vi "DCTOpticalSwitch.vi"() -> ()   [LabVIEW 2011]
uses:
  Dependencies/DCS/flex05-4chPascal.dll
  Dependencies/DCS/flex05oem8chautoPASCAL.dll
  Dependencies/Zaber/Zaber A Series.lvlib
panel:
  in  "Start Program":bool
  in  "DAQ Port":tag
  in  "Raster X Reverse":bool=TRUE
  in  "Max speed (mm/s)":dbl=35.0
  in  "Microstep resolution":dbl=0.124023437
  in  "Close":bool
  in  "Optical Output":T1
  in  "Optical Input":T2
  out "Detector Indicator":T3 {"Det 8" format="%.3f"; "Det 7" format="%.3f"; "Det 6" format="%.3f"; "Det 5" format="%.3f"; "Det 4" format="%.3f"; "Det 3" format="%.3f"; "Det 2 2" format="%.3f"; "Det 1" format="%.3f"}
  in  "Detector\n Buttons":T4
  out "Y-axis Device":string
  out "X-axis Device":string
  out "Y Index":i32
  out "X Index":i32
  in  "Update Time (ms):":u32=44
  out "Computer time":string
  out "Time Left (ms)":sgl format="%.3f"
  in  "Duration Time (ms):":sgl=2000.0
  out "Y Position [mm]":dbl
  out "X Position [mm]":dbl
  in  "Stage Controls Tabs":enum32{"Raster Scan", "Manual"}(tab) caption="Stage Controls"
  out "Raster Scanning":bool
  in  "X Steps":i32
  in  "Y Steps":i32
  in  "Y Increment [mm]":dbl
  in  "X Increment [mm]":dbl
  out "Y Total Distance [mm]":dbl
  out "X Total Distance [mm]":dbl
  in  "Raster Scan":bool
  out "Scanning":bool
  in  "Move X":bool
  in  "Move Y":bool
  in  "Home":bool
  in  "Scan":bool
  in  "Number of Scans":i32=1 min=1
  in  "X distance [mm]":dbl
  in  "Y distance  [mm]":dbl
  in  "File Name:":string="AAA"
  in  "File Path:":path=path "C:/Users/aproctor1/Desktop/Our Attempts/DCS practice data"
  in  "Clear Plots":bool
  out "g2":cluster{"Delay Time":sgl[], sgl[]}[](graph) caption="Normalized Correlation Function"
  out "Tau":T5(graph)={"[0]"=0.0, "[1]"=1.0, "[2]"=2.0, "[3]"=3.0, "[4]"=4.0, "[5]"=5.0, "[6]"=6.0, "[7]"=7.0, "[8]"=8.0} caption="Relative changes of flow"
  in  "Detectors Select":enum32{"4 Detectors", "8 Detectors"}(radio)
  in  "Stage Port":refnum<visa-resource-name>="COM8"
  # "DCS Control Panel"
  # "Optical Switch"
  # "Stage Control"
  # "Probe Location"
  # "Instructions: \n1. Initialize the following settings first: (these will be locked later)\n      - Detectors Select\n      - DAQ Port (port 0 for NI USB 6001)\n      - Optical Switch Inputs and Outputs\n      - Stage Port (for Zaber)\n2. Click on \"Start Program\" which will lock the above settings and enable stage controls\n3. When settings from step 1 are locked, input options for raster scanning or manual scanning\n4. Free to do whatever \n5. Close the program by clicking the close button"
  # "Max Distance: 203.2 mm"
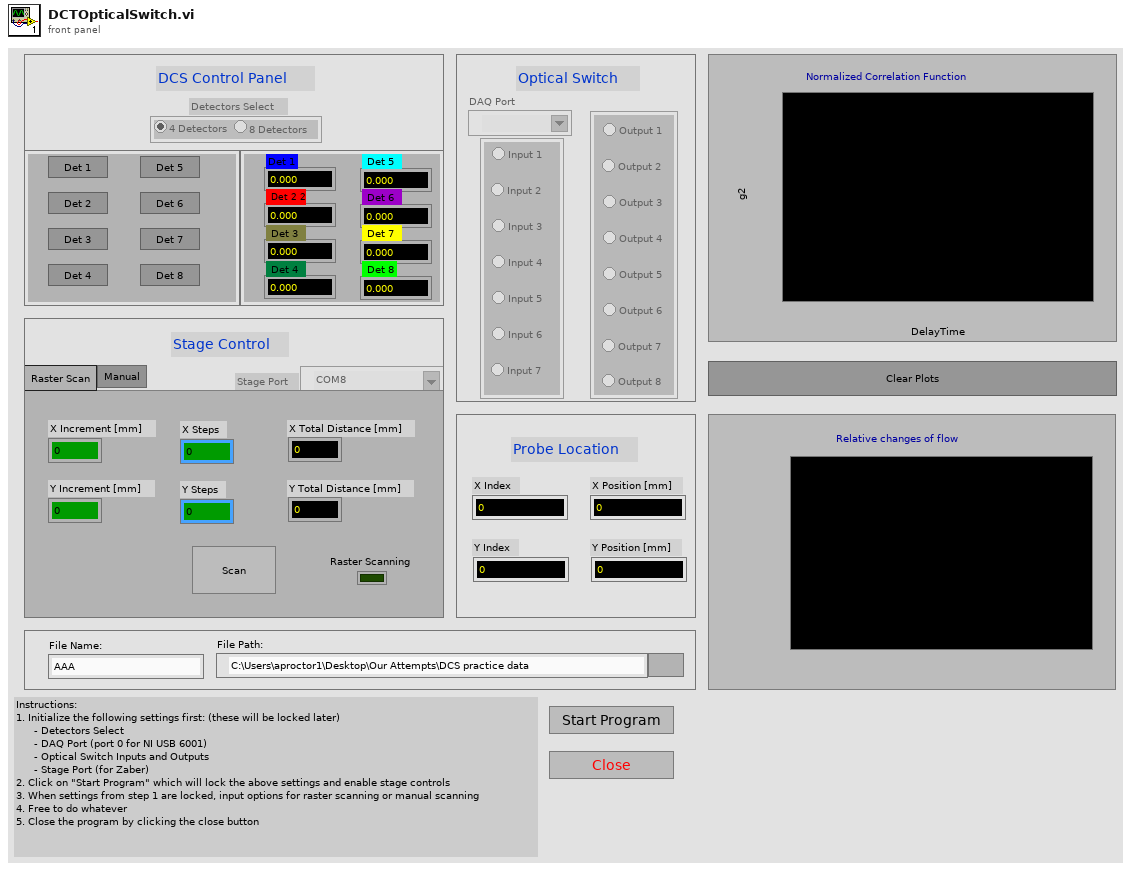
[diagram p1: front panel]
types:
  T1 = cluster{"Output 1":bool, "Output 2":bool, "Output 3":bool, "Output 4":bool, "Output 5":bool, "Output 6":bool, "Output 7":bool, "Output 8":bool}
  T2 = cluster{"Input 1":bool, "Input 2":bool, "Input 3":bool, "Input 4":bool, "Input 5":bool, "Input 6":bool, "Input 7":bool}
  T3 = cluster{"Det 1":sgl, " Det 2 2":sgl, " Det 3":sgl, " Det 4":sgl, " Det 5":sgl, " Det 6":sgl, " Det 7":sgl, " Det 8":sgl}
  T4 = cluster{"btnDet 1":bool, "btnDet 2":bool, "btnDet 3":bool, "btnDet 4":bool, "btnDet 5":bool, "btnDet 6":bool, "btnDet 7":bool, "btnDet 8":bool}
  T5 = cluster{"[0]":dbl, "[1]":dbl, "[2]":dbl, "[3]":dbl, "[4]":dbl, "[5]":dbl, "[6]":dbl, "[7]":dbl, "[8]":dbl}
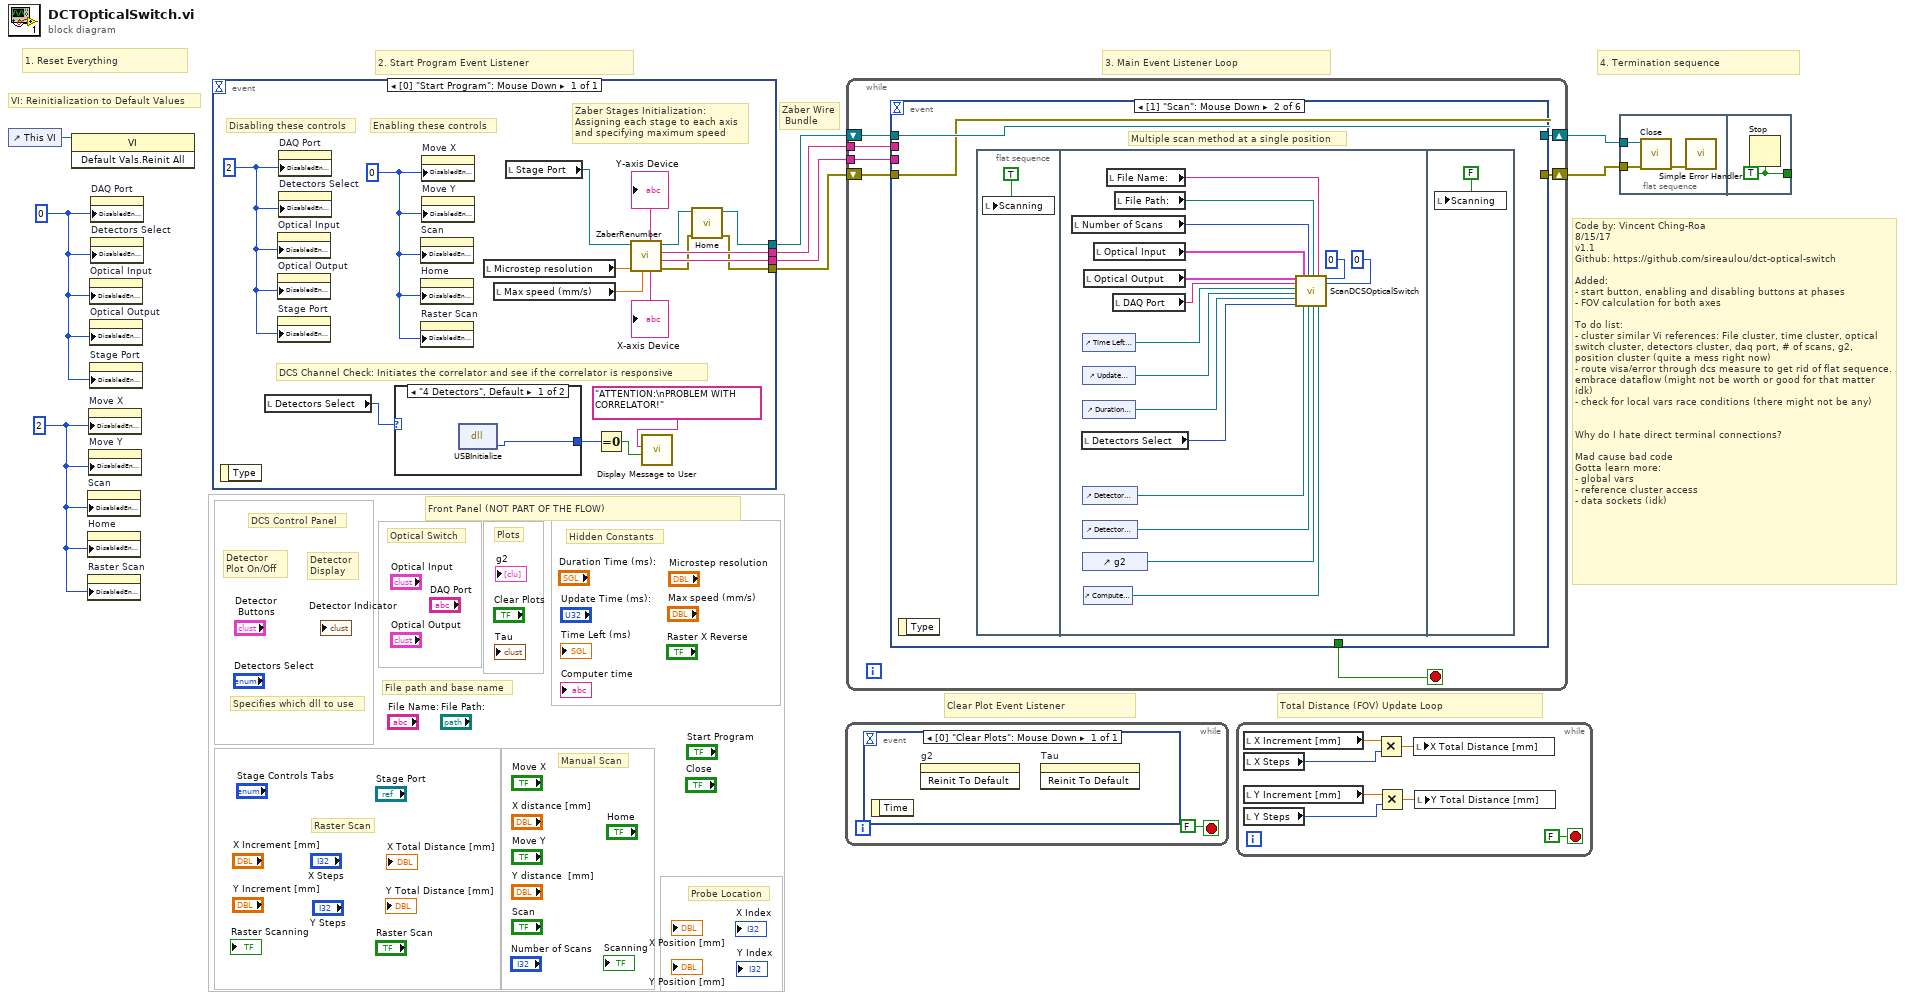
[diagram p0: block diagram]
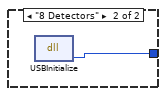
[diagram p2: hidden frame]
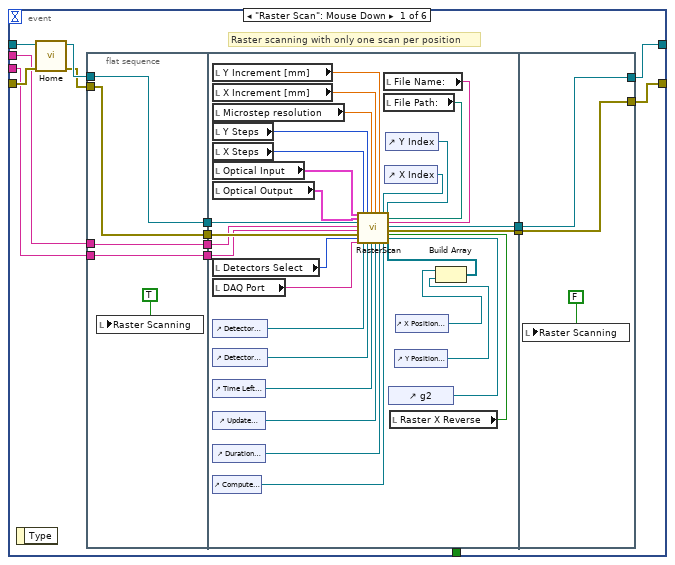
[diagram p3: hidden frame]
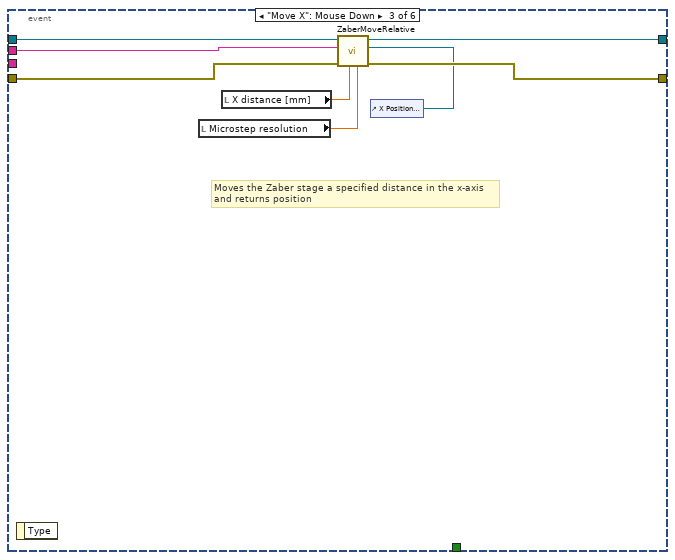
[diagram p4: hidden frame]
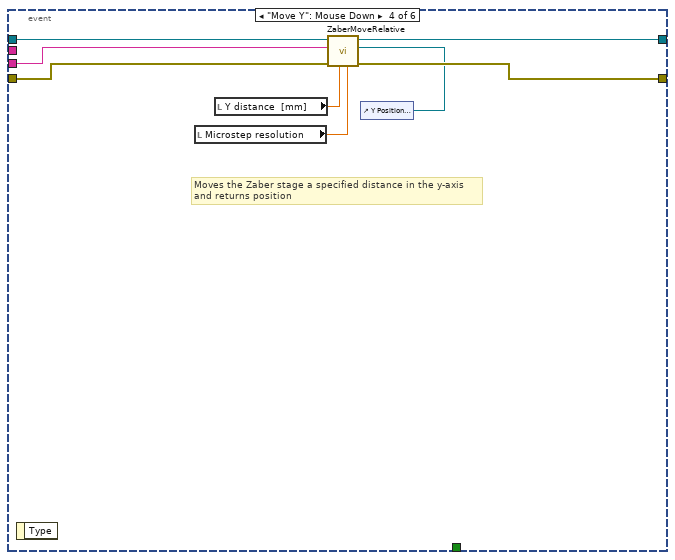
[diagram p5: hidden frame]
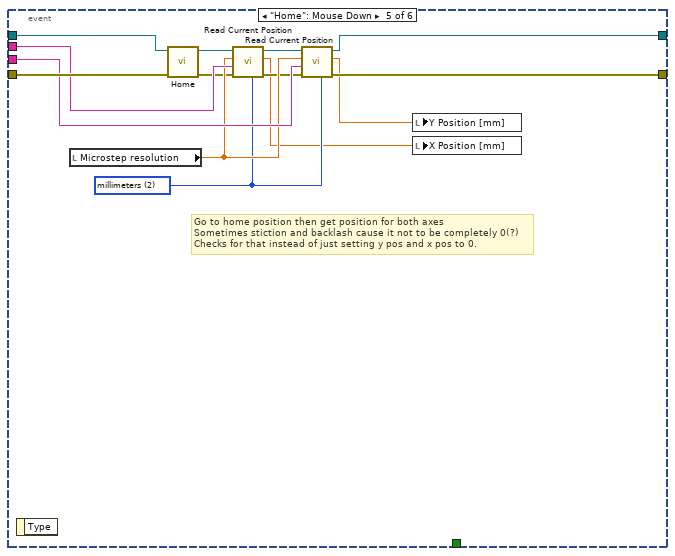
[diagram p6: hidden frame]
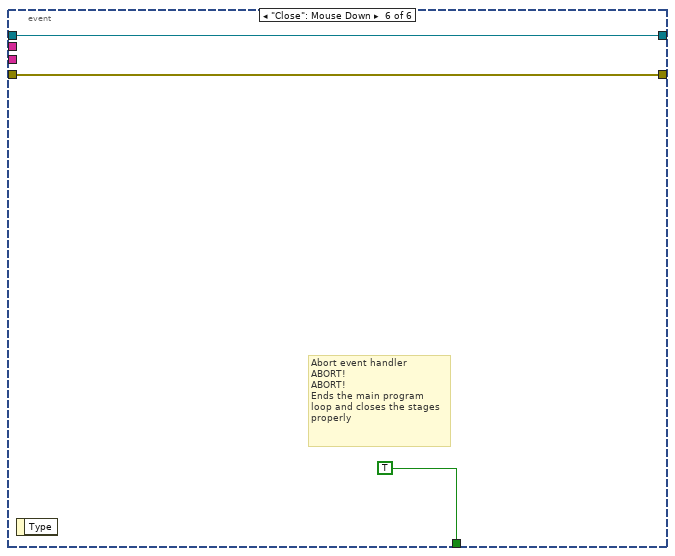
[diagram p7: hidden frame]
diagram:
  w1 = 2
  w2 = 0
  # "Total Distance (FOV) Update Loop"
  # "1. Reset Everything"
  # "2. Start Program Event Listener"
  # "Code by: Vincent Ching-Roa\n8/15/17\nv1.1\nGithub: https://github.com/sireaulou/dct-optical-switch\n\nAdded:\n- start button, enabling and disabling buttons at phases\n- FOV calculation for both axes \n\nTo do list:\n- cluster similar Vi references: File cluster, time cluster, optical switch cluster, detectors cluster, daq port, # of scans, g2, position cluster (quite a mess right now)\n- route visa/error through dcs measure to get rid of flat sequence. embrace dataflow (might not be worth or good for that matter idk)\n- check for local vars race conditions (there might not be any)\n\n\nWhy do I hate direct terminal connections?\n\nMad cause bad code\nGotta learn more:\n- global vars\n- reference cluster access\n- data sockets (idk)"
  # "4. Termination sequence"
  # "Clear Plot Event Listener"
  # "Zaber Wire\n Bundle"
  # "3. Main Event Listener Loop"
  # "VI: Reinitialization to Default Values"
  # "Front Panel (NOT PART OF THE FLOW)"
  # "Specifies which dll to use"
  # "Hidden Constants"
  # "Plots"
  # "File path and base name"
  # "Probe Location"
  # "Manual Scan"
  # "Raster Scan"
  # "Optical Switch"
  # "Detector \nDisplay"
  # "Detector\nPlot On/Off"
  # "DCS Control Panel"
  n1 = control-ref of="This VI"() -> (w9:refnum<vi>)
  n2 = invoke class="VI" method="Default Vals.Reinit All"(reference=w9) -> ()  [unwired: 2 in, 3 out]
  n3 = property on="Scan" class="Bool (strict)"("DisabledEnum"=w1) -> ()  [unwired: 2 in, 2 out]
  n4 = property on="Home" class="Bool (strict)"("DisabledEnum"=w1) -> ()  [unwired: 2 in, 2 out]
  n5 = property on="Raster Scan" class="Bool (strict)"("DisabledEnum"=w1) -> ()  [unwired: 2 in, 2 out]
  n6 = property on="Move X" class="Bool (strict)"("DisabledEnum"=w1) -> ()  [unwired: 2 in, 2 out]
  n7 = property on="Move Y" class="Bool (strict)"("DisabledEnum"=w1) -> ()  [unwired: 2 in, 2 out]
  n8 = property on="Optical Input" class="Clust (strict)"("DisabledEnum"=w2) -> ()  [unwired: 2 in, 2 out]
  n9 = property on="Optical Output" class="Clust (strict)"("DisabledEnum"=w2) -> ()  [unwired: 2 in, 2 out]
  n10 = property on="Stage Port" class="VISAName"("DisabledEnum"=w2) -> ()  [unwired: 2 in, 2 out]
  n11 = property on="DAQ Port" class="DAQmxName"("DisabledEnum"=w2) -> ()  [unwired: 2 in, 2 out]
  n12 = property on="Detectors Select" class="RadioBtnsControl (strict)"("DisabledEnum"=w2) -> ()  [unwired: 2 in, 2 out]
  n13 = event shown="[0] \"Start Program\": Mouse Down" {
    selector: _ -> [_]
    dyn-events: _ -> [_]
    timeout: _ -> [_]
    tunnel: [w19] -> w8
    tunnel: [w18] -> w7
    tunnel: [w14] -> w4
    tunnel: [w12] -> w3
    event "Start Program": Mouse Down {
      w10 = 0
      w11 = 2
      # "Enabling these controls"
      # "Disabling these controls"
      # "Zaber Stages Initialization:\nAssigning each stage to each axis\nand specifying maximum speed"
      # "DCS Channel Check: Initiates the correlator and see if the correlator is responsive"
      n14 = event-data() -> ()  [unwired: 1 in, 1 out]
      n15 = local read "Detectors Select"() -> (w23:enum32{"4 Detectors", "8 Detectors"})
      n16 = property on="Optical Input" class="Clust (strict)"("DisabledEnum"=w11) -> ()  [unwired: 2 in, 2 out]
      n17 = property on="Optical Output" class="Clust (strict)"("DisabledEnum"=w11) -> ()  [unwired: 2 in, 2 out]
      n18 = property on="Stage Port" class="VISAName"("DisabledEnum"=w11) -> ()  [unwired: 2 in, 2 out]
      n19 = property on="DAQ Port" class="DAQmxName"("DisabledEnum"=w11) -> ()  [unwired: 2 in, 2 out]
      n20 = property on="Detectors Select" class="RadioBtnsControl (strict)"("DisabledEnum"=w11) -> ()  [unwired: 2 in, 2 out]
      n21 = case shown="\"4 Detectors\", Default" w23 {
        tunnel: [w27 w28] -> w26
        frame "4 Detectors", Default {
          n22 = dll-call lib="C:/LABVIEWcodesWorksInC/UnderDeveopmentNeedChecking/Vincent2017/DCTOpticalSwitch/Dependencies/DCS/flex05-4chPascal.dll" fn="USBInitialize"() -> ("return type"=w27:u8)  [unwired: 3 in, 2 out]
        }
        frame "8 Detectors" {
          n23 = dll-call lib="C:/LABVIEWcodesWorksInC/UnderDeveopmentNeedChecking/Vincent2017/DCTOpticalSwitch/Dependencies/DCS/flex05oem8chautoPASCAL.dll" fn="USBInitialize"() -> ("return type"=w28:u8)  [unwired: 3 in, 2 out]
        }
      }
      n24 = property on="Scan" class="Bool (strict)"("DisabledEnum"=w10) -> ()  [unwired: 2 in, 2 out]
      n25 = property on="Home" class="Bool (strict)"("DisabledEnum"=w10) -> ()  [unwired: 2 in, 2 out]
      n26 = property on="Raster Scan" class="Bool (strict)"("DisabledEnum"=w10) -> ()  [unwired: 2 in, 2 out]
      n27 = property on="Move X" class="Bool (strict)"("DisabledEnum"=w10) -> ()  [unwired: 2 in, 2 out]
      n28 = property on="Move Y" class="Bool (strict)"("DisabledEnum"=w10) -> ()  [unwired: 2 in, 2 out]
      n29 = local read "Microstep resolution"() -> (w17:dbl)
      n30 = local read "Max speed (mm/s)"() -> (w16:dbl)
      n31 = local read "Stage Port"() -> (w21:refnum<visa-resource-name>)
      n32 = Equal To 0?(x=w26) -> (x = 0?=w24:bool)
      n33 = call "ZaberRenumber.vi"("max speed (mm/s)"=w16, "resolution"=w17, "VISA Refnum in"=w21) -> ("error out"=w13:errorcluster, "Device 1"=w18:string, "Device 0"=w19:string, "VISA Refnum out"=w15:refnum<visa-resource-name>, "X-axis Device"=→"X-axis Device":string, "Y-axis Device"=→"Y-axis Device":string)  [unwired: 3 in]
      n34 = call "Display Message to User"("Enable"=w24, "Message"="ATTENTION:\nPROBLEM WITH CORRELATOR!") -> ()  [unwired: 8 in, 2 out]
      n35 = call "Home.vi"("error in (no error)"=w13, "VISA resource name"=w15) -> ("error out"=w12:errorcluster, "VISA resource name out"=w14:refnum<visa-resource-name>)  [unwired: 8 in]
    }
  }
  n36 = while {
    stop <- FALSE stop-if-true
    n37 = event shown="[0] \"Clear Plots\": Mouse Down" {
      selector: _ -> [_]
      dyn-events: _ -> [_]
      timeout: _ -> [_]
      event "Clear Plots": Mouse Down {
        n38 = event-data() -> ()  [unwired: 1 in, 1 out]
        n39 = invoke on="g2" class="XYGraph (strict)" method="Reinit To Default"() -> ()  [unwired: 3 in, 3 out]
        n40 = invoke on="Tau" class="WFChart (strict)" method="Reinit To Default"() -> ()  [unwired: 3 in, 3 out]
      }
    }
  }
  n41 = while {
    shift-right: [w34] -> w6
    shift-left: w4 -> [w32]
    shift-right: [w33] -> w5
    shift-left: w3 -> [w31]
    tunnel: w8 -> [w36]
    tunnel: w7 -> [w35]
    stop <- w30 stop-if-true
    n42 = event shown="[1] \"Scan\": Mouse Down" {
      selector: _ -> [_ _ _ _ _ _]
      dyn-events: _ -> [_ _ _ _ _ _]
      timeout: _ -> [_ _ _ _ _ _]
      tunnel: w32 -> [w50 w90 w115 w124 w138 w140]
      tunnel: w36 -> [w44 _ w116 _ w136 _]
      tunnel: w35 -> [w43 _ _ w118 w135 _]
      tunnel: w31 -> [w49 w89 w112 w121 w137 w139]
      tunnel: [w38 w90 w114 w123 w129 w140] -> w34
      tunnel: [w37 w89 w113 w122 w130 w139] -> w33
      tunnel: [_ _ _ _ _ TRUE] -> w30
      event "Raster Scan": Mouse Down {
        # "Raster scanning with only one scan per position"
        n43 = event-data() -> ()  [unwired: 1 in, 1 out]
        n44 = call "Home.vi"("error in (no error)"=w49, "VISA resource name"=w50) -> ("error out"=w46:errorcluster, "VISA resource name out"=w47:refnum<visa-resource-name>)  [unwired: 8 in]
        n45 = flat-sequence {
          tunnel: [w54] -> w48
          tunnel: w47 -> [w54]
          tunnel: w46 -> [w53]
          tunnel: [w53] -> w45
          tunnel: w44 -> [w52]
          tunnel: w43 -> [w51]
          tunnel: [w52] -> w42
          tunnel: [w51] -> w41
          tunnel: w48 -> [w78]
          tunnel: w45 -> [w77]
          tunnel: w42 -> [w76]
          tunnel: w41 -> [w75]
          tunnel: [w64] -> w40
          tunnel: [w63] -> w39
          tunnel: w40 -> [w86]
          tunnel: w39 -> [w87]
          tunnel: [w87] -> w38
          tunnel: [w86] -> w37
          frame #0 {
            n46 = local write "Raster Scanning"(TRUE) -> ()
          }
          frame #1 {
            n47 = local read "Y Increment [mm]"() -> (w85:dbl)
            n48 = local read "X Increment [mm]"() -> (w84:dbl)
            n49 = local read "Microstep resolution"() -> (w83:dbl)
            n50 = local read "Y Steps"() -> (w82:i32)
            n51 = local read "X Steps"() -> (w81:i32)
            n52 = local read "Optical Input"() -> (w80:T2)
            n53 = local read "Optical Output"() -> (w79:T1)
            n54 = local read "Detectors Select"() -> (w74:enum32{"4 Detectors", "8 Detectors"})
            n55 = local read "DAQ Port"() -> (w73:tag)
            n56 = control-ref of="Detector Buttons"() -> (w72:refnum<vi>)
            n57 = control-ref of="Detector Indicator"() -> (w71:refnum<vi>)
            n58 = control-ref of="Time Left (ms)"() -> (w70:refnum<vi>)
            n59 = control-ref of="Update Time (ms):"() -> (w69:refnum<vi>)
            n60 = control-ref of="Duration Time (ms):"() -> (w68:refnum<vi>)
            n61 = control-ref of="Computer time"() -> (w67:refnum<vi>)
            n62 = local read "File Name:"() -> (w62:string)
            n63 = local read "File Path:"() -> (w61:path)
            n64 = control-ref of="X Index"() -> (w60:refnum<vi>)
            n65 = control-ref of="Y Index"() -> (w59:refnum<vi>)
            n66 = control-ref of="g2"() -> (w66:refnum<vi>)
            n67 = local read "Raster X Reverse"() -> (w65:bool)
            n68 = control-ref of="Y Position [mm]"() -> (w58:refnum<vi>)
            n69 = control-ref of="X Position [mm]"() -> (w57:refnum<vi>)
            n70 = Build Array(w57, w58) -> (w56:refnum<vi>[])
            n71 = call "RasterScan.vi"("Optical Input"=w80, "Optical Output"=w79, "Stage Port"=w78, "x-axis stage"=w76, "y-axis stage"=w75, "error in (no error)"=w77, "Detectors Select"=w74, "DAQ Port"=w73, "X Steps"=w81, "Detector Buttons"=w72, "Y Steps"=w82, "Detector Indicator"=w71, "Microstep resolution"=w83, "Time Left (ms)"=w70, "X Increment [mm]"=w84, "Update Time (ms):"=w69, "Y Increment [mm]"=w85, "Duration Time (ms):"=w68, "x index"=w60, "Computer time"=w67, "y index"=w59, "File Path:"=w61, "File Name:"=w62, "Raster X Reverse"=w65, "g2"=w66, "Position array"=w56) -> ("VISA Refnum out"=w63:refnum<visa-resource-name>, "error out"=w64:errorcluster)
          }
          frame #2 {
            n72 = local write "Raster Scanning"(FALSE) -> ()
          }
        }
      }
      event "Scan": Mouse Down {
        # "Multiple scan method at a single position"
        n73 = event-data() -> ()  [unwired: 1 in, 1 out]
        n74 = flat-sequence {
          frame #0 {
            n75 = local write "Scanning"(TRUE) -> ()
          }
          frame #1 {
            n76 = local read "Number of Scans"() -> (w105:i32)
            n77 = local read "Detectors Select"() -> (w98:enum32{"4 Detectors", "8 Detectors"})
            n78 = control-ref of="Time Left (ms)"() -> (w101:refnum<vi>)
            n79 = control-ref of="Update Time (ms):"() -> (w100:refnum<vi>)
            n80 = control-ref of="Duration Time (ms):"() -> (w99:refnum<vi>)
            n81 = control-ref of="Detector\n Buttons"() -> (w97:refnum<vi>)
            n82 = control-ref of="Detector Indicator"() -> (w96:refnum<vi>)
            n83 = control-ref of="g2"() -> (w95:refnum<vi>)
            n84 = local read "Optical Output"() -> (w103:T1)
            n85 = control-ref of="Computer time"() -> (w94:refnum<vi>)
            n86 = local read "Optical Input"() -> (w104:T2)
            n87 = local read "File Name:"() -> (w107:string)
            n88 = local read "DAQ Port"() -> (w102:tag)
            n89 = local read "File Path:"() -> (w106:path)
            n90 = call "ScanDCSOpticalSwitch.vi"("Optical Output"=w103, "DAQ Port"=w102, "Time Left (ms)"=w101, "Update Time (ms):"=w100, "Duration Time (ms):"=w99, "Detectors Select"=w98, "Optical Input"=w104, "Detector\n Buttons"=w97, "Number of Scans"=w105, "Detector Indicator"=w96, "File Path:"=w106, "g2"=w95, "File Name:"=w107, "Computer time"=w94, "X index"=0, "Y index"=0) -> ()  [unwired: 4 in]
          }
          frame #2 {
            n91 = local write "Scanning"(FALSE) -> ()
          }
        }
      }
      event "Move X": Mouse Down {
        # "Moves the Zaber stage a specified distance in the x-axis\nand returns position"
        n92 = event-data() -> ()  [unwired: 1 in, 1 out]
        n93 = local read "Microstep resolution"() -> (w110:dbl)
        n94 = local read "X distance [mm]"() -> (w111:dbl)
        n95 = control-ref of="X Position [mm]"() -> (w109:refnum<vi>)
        n96 = call "ZaberMoveRelative.vi"("Position Indicator"=w109, "Microstep resolution"=w110, "distance [mm]"=w111, "error in (no error)"=w112, "Device"=w116, "VISA Refnum in"=w115) -> ("error out"=w113:errorcluster, "VISA Refnum out"=w114:refnum<visa-resource-name>)  [unwired: 4 in]
      }
      event "Move Y": Mouse Down {
        # "Moves the Zaber stage a specified distance in the y-axis \nand returns position"
        n97 = event-data() -> ()  [unwired: 1 in, 1 out]
        n98 = local read "Microstep resolution"() -> (w119:dbl)
        n99 = local read "Y distance  [mm]"() -> (w120:dbl)
        n100 = control-ref of="Y Position [mm]"() -> (w117:refnum<vi>)
        n101 = call "ZaberMoveRelative.vi"("Position Indicator"=w117, "Microstep resolution"=w119, "distance [mm]"=w120, "error in (no error)"=w121, "Device"=w118, "VISA Refnum in"=w124) -> ("error out"=w122:errorcluster, "VISA Refnum out"=w123:refnum<visa-resource-name>)  [unwired: 4 in]
      }
      event "Home": Mouse Down {
        w127 = u16 2 items=["microsteps", "microns", "millimeters", "inches"] ("Units (0: microsteps)")
        # "Go to home position then get position for both axes\nSometimes stiction and backlash cause it not to be completely 0(?)\nChecks for that instead of just setting y pos and x pos to 0."
        n102 = event-data() -> ()  [unwired: 1 in, 1 out]
        n103 = local read "Microstep resolution"() -> (w132:dbl)
        n104 = call "Home.vi"("error in (no error)"=w137, "VISA resource name"=w138) -> ("error out"=w128:errorcluster, "VISA resource name out"=w134:refnum<visa-resource-name>)  [unwired: 8 in]
        n105 = call "Read Current Position.vi"("Units (0: microsteps)"=w127, "error in (no error)"=w128, "Device and Axis"=w136, "Microstep Size (0)"=w132, "VISA resource name"=w134) -> ("error out"=w131:errorcluster, "Position"=w126:dbl, "VISA resource name out"=w133:refnum<visa-resource-name>)  [unwired: 4 in]
        n106 = call "Read Current Position.vi"("Units (0: microsteps)"=w127, "error in (no error)"=w131, "Device and Axis"=w135, "Microstep Size (0)"=w132, "VISA resource name"=w133) -> ("error out"=w130:errorcluster, "Position"=w125:dbl, "VISA resource name out"=w129:refnum<visa-resource-name>)  [unwired: 4 in]
        n107 = local write "Y Position [mm]"(w125) -> ()
        n108 = local write "X Position [mm]"(w126) -> ()
      }
      event "Close": Mouse Down {
        # "Abort event handler\nABORT!\nABORT!\nEnds the main program\nloop and closes the stages\nproperly"
        n109 = event-data() -> ()  [unwired: 1 in, 1 out]
      }
    }
  }
  n110 = while {
    stop <- FALSE stop-if-true
    n111 = local read "X Increment [mm]"() -> (w147:dbl)
    n112 = local read "X Steps"() -> (w146:i32)
    n113 = local read "Y Increment [mm]"() -> (w144:dbl)
    n114 = local read "Y Steps"() -> (w143:i32)
    n115 = Multiply(x=w147, y=w146) -> (x*y=w145:dbl)
    n116 = Multiply(x=w144, y=w143) -> (x*y=w142:dbl)
    n117 = local write "X Total Distance [mm]"(w145) -> ()
    n118 = local write "Y Total Distance [mm]"(w142) -> ()
  }
  n119 = flat-sequence {
    tunnel: w6 -> [w151]
    tunnel: w5 -> [w150]
    tunnel: [w152] -> _
    frame #0 {
      n120 = call "Close.vi"("error in (no error)"=w150, "VISA resource name"=w151) -> ("error out"=w149:errorcluster)  [unwired: 9 in]
      n121 = call <vilib>:"Simple Error Handler.vi"("error in (no error)"=w149) -> ()  [unwired: 4 in, 5 out]
    }
    frame #1 {
      w152 = TRUE
      n122 = Stop(stop? (T)=w152) -> ()
    }
  }
